vi "fitresultmaker.vi"(10 "best fit parameter":dbl[](array[numeric]), 11 "num of gaussian peaks":i32) -> (3 "FIT RESULTS":T1(array[cluster]))   [LabVIEW 2020]
panel:
  in  "GAUSSIAN CLUSTER":T2
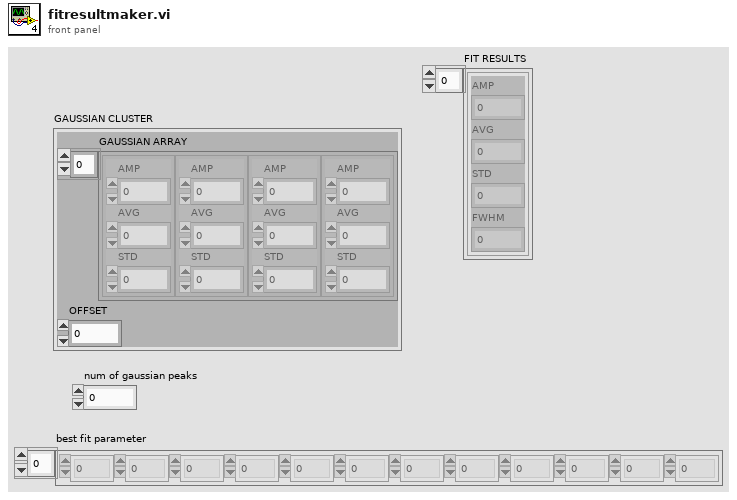
[diagram p1: front panel]
types:
  T1 = cluster{"AMP":dbl, "AVG":dbl, "STD":dbl, "FWHM":dbl}[]
  T2 = cluster{"GAUSSIAN ARRAY":cluster{"AMP":dbl, "AVG":dbl, "STD":dbl}[], "OFFSET":dbl}
  T3 = cluster{"AMP":dbl, "AVG":dbl, "STD":dbl, "FWHM":dbl}
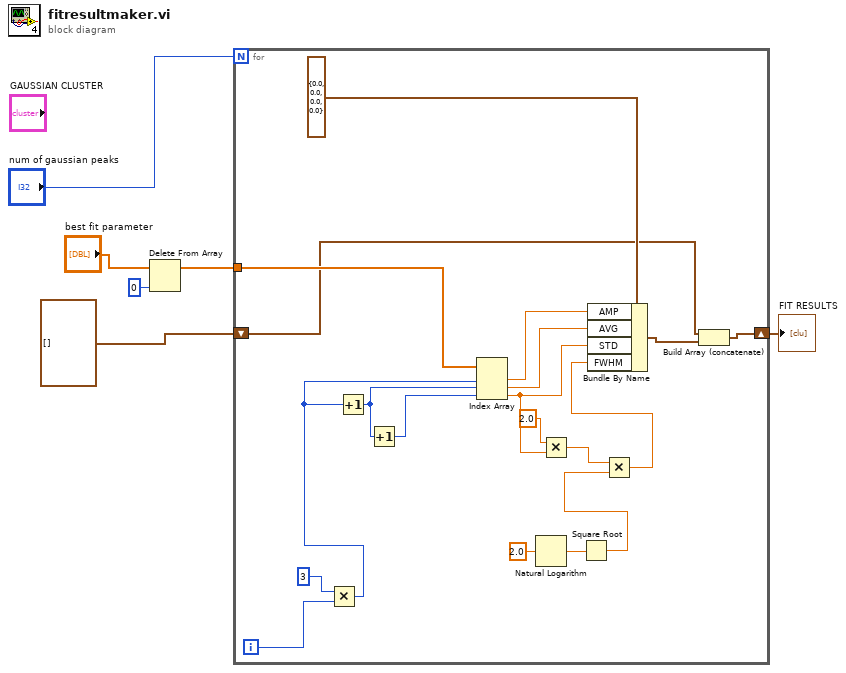
[diagram p0: block diagram]
diagram:
  n1 = Delete From Array(array="best fit parameter", index=0) -> (array with subset deleted=w2:dbl[])  [unwired: 1 in, 1 out]
  n2 = for {
    N: "num of gaussian peaks" -> [_]
    shift-right: [w14] -> w1
    shift-left: T1 [] ("GAUSSIAN ARRAY") -> [w15]
    tunnel: w2 -> [w19]
    i -> [w23]
    n3 = Multiply(x=3, y=w23) -> (x*y=w22:i32)
    n4 = Increment(x=w22) -> (x+1=w21:i32)
    n5 = Increment(x=w21) -> (x+1=w20:i32)
    n6 = Index Array(array=w19, index #1=w22, index #2=w21, index #3=w20) -> (element #1=w18:dbl, element #2=w17:dbl, element #3=w13:dbl)
    n7 = Natural Logarithm(1:2.0 ("x")) -> (0:w9:dbl)
    n8 = Multiply(x=2.0, y=w13) -> (x*y=w11:dbl)
    n9 = Square Root(x=w9) -> (sqrt(x)=w8:dbl)
    n10 = Multiply(x=w11, y=w8) -> (x*y=w7:dbl)
    n11 = Bundle By Name(cluster=T3 {"AMP"=0.0, "AVG"=0.0, "STD"=0.0, "FWHM"=0.0} ("GAUSSIAN"), "AMP"=w18, "AVG"=w17, "STD"=w13, "FWHM"=w7) -> (w16:T3)
    n12 = Build Array (concatenate)(w15, w16) -> (w14:T1)
  }
  "FIT RESULTS" <- w1
